vi "Command.vi"(7 "no read (false)":bool, 8 "error in (no error)":errorcluster, 9 "command payload":u8[](array[numeric]), 10 "command":u8, 11 "TroSpec in":refnum<class "PL ISTEQ TroSpec.lvclass">) -> (0 "error out":errorcluster, 2 "response payload":u8[](array[numeric]), 3 "TroSpec out":refnum<class "PL ISTEQ TroSpec.lvclass">)   [LabVIEW 2015, in "PL ISTEQ TroSpec.lvclass"]
doc: "Sends command and returns response payload if <b>no read</b> is not selected."
uses:
  PL ISTEQ TroSpec.lvclass
  PL ISTEQ TroSpec.lvclass/PL ISTEQ TroSpec.ctl
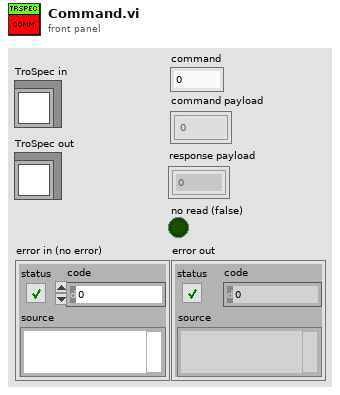
[diagram p1: front panel]
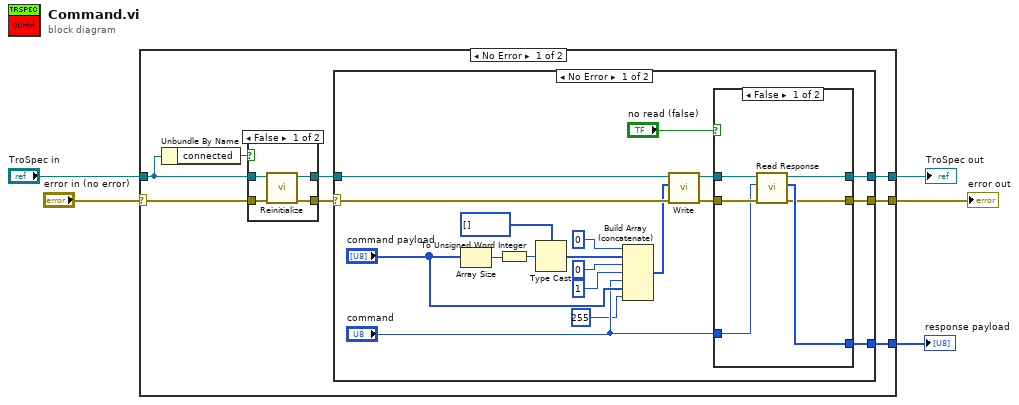
[diagram p0: block diagram]
diagram:
  n1 = case shown="No Error" "error in (no error)" {
    selector: "error in (no error)" -> [w11 w50]
    tunnel: "TroSpec in" -> [w12 w49]
    tunnel: [w8 w50] -> w4
    tunnel: [w7 w49] -> w2
    tunnel: [w6 _] -> w1
    frame No Error {
      n2 = Unbundle By Name(w12) -> ("connected"=w13:bool)
      n3 = case shown="False" w13 {
        tunnel: w12 -> [w46 w48]
        tunnel: w11 -> [w45 w47]
        tunnel: [w44 w48] -> w9
        tunnel: [w43 w47] -> w10
        frame False {
          n4 = call "Reinitialize.vi"("error in (no error)"=w45, "TroSpec in"=w46) -> ("error out"=w43:errorcluster, "TroSpec out"=w44:refnum<class "PL ISTEQ TroSpec.lvclass">)  [unwired: 8 in]
        }
        frame True {
        }
      }
      n5 = case shown="No Error" w10 {
        selector: w10 -> [w21 w42]
        tunnel: w9 -> [w22 w41]
        tunnel: [w32 w42] -> w8
        tunnel: [w31 w41] -> w7
        tunnel: [w15 _] -> w6
        frame No Error {
          n6 = Array Size(array="command payload") -> (size(s)=w23:i32)
          n7 = To Unsigned Word Integer(number=w23) -> (unsigned 16bit integer=w24:u16)
          n8 = Type Cast(type=u8[] [] ("command payload"), x=w24) -> (*(type *) &x=w26:u8[])
          n9 = Build Array (concatenate)(u8 0 ("element"), w26, u8 0 ("command"), u8 1 ("command"), "command", "command payload", u8 255 ("command")) -> (w20:u8[])
          n10 = call "Write.vi"("error in (no error)"=w21, "data"=w20, "TroSpec in"=w22) -> ("error out"=w18:errorcluster, "TroSpec out"=w19:refnum<class "PL ISTEQ TroSpec.lvclass">)  [unwired: 7 in]
          n11 = case shown="False" "no read (false)" {
            tunnel: [w34 w39] -> w32
            tunnel: [w33 w40] -> w31
            tunnel: w19 -> [w38 w40]
            tunnel: w18 -> [w37 w39]
            tunnel: "command" -> [w36 _]
            tunnel: [w35 _] -> w15
            frame False {
              n12 = call "Read Response.vi"("error in (no error)"=w37, "command"=w36, "TroSpec in"=w38) -> ("error out"=w34:errorcluster, "response payload"=w35:u8[], "TroSpec out"=w33:refnum<class "PL ISTEQ TroSpec.lvclass">)  [unwired: 6 in]
            }
            frame True {
            }
          }
        }
        frame Error {
        }
      }
    }
    frame Error {
    }
  }
  "error out" <- w4
  "TroSpec out" <- w2
  "response payload" <- w1
